vi "Wait for Control Panel Start.vi"(8 "error in (no error)":errorcluster, 10 "timeout in ms (-1)":i32=-1, 11 "Generic Controller in":refnum<class "Generic Plugin.lvclass">) -> (0 "error out":errorcluster, 2 "Timeout?":bool, 3 "Generic Controller out":refnum<class "Generic Plugin.lvclass">)   [LabVIEW 2020, in "Generic Plugin.lvclass"]
doc: "Wait for a message indicating that the control panel has started, or timeout if a value is given for the wait time."
uses:
  Generic Plugin.lvclass
  Generic Plugin.lvclass/Generic Plugin.ctl
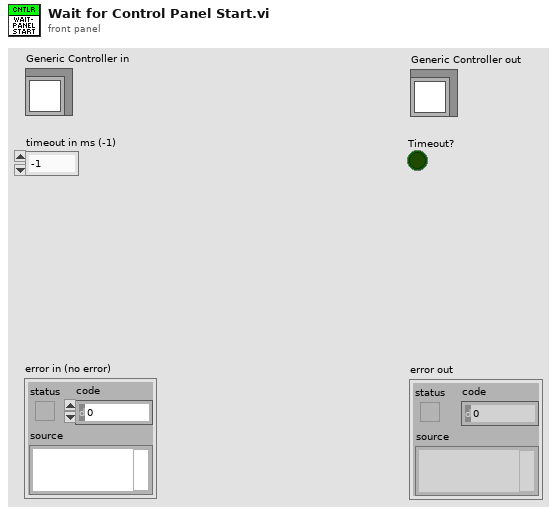
[diagram p1: front panel]
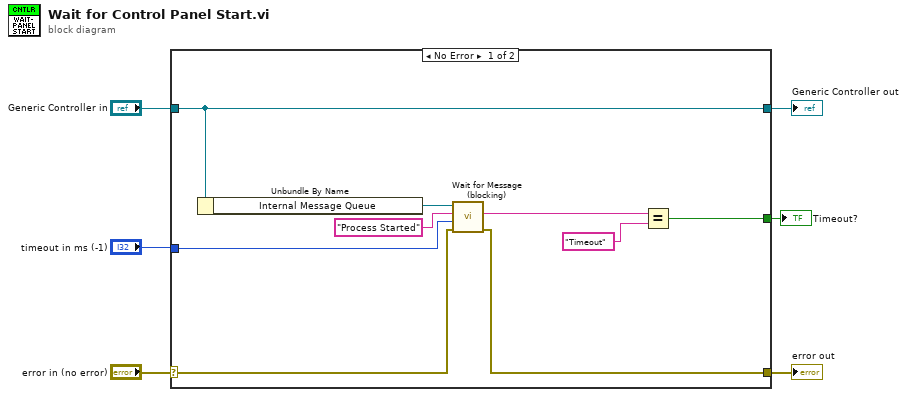
[diagram p0: block diagram]
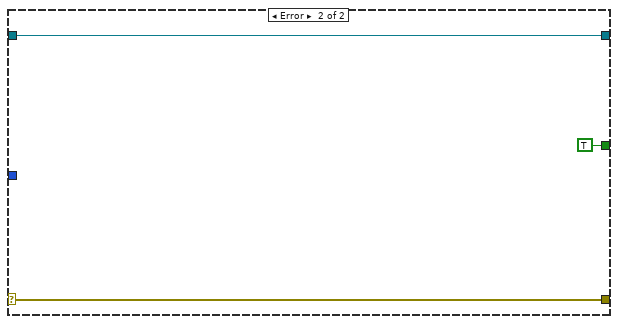
[diagram p2: hidden frame]
diagram:
  n1 = case shown="No Error" "error in (no error)" {
    selector: "error in (no error)" -> [w13 w18]
    tunnel: [w11 w18] -> w5
    tunnel: [w15 w17] -> w3
    tunnel: "Generic Controller in" -> [w15 w17]
    tunnel: "timeout in ms (-1)" -> [w10 _]
    tunnel: [w7 TRUE] -> w1
    frame No Error {
      n2 = Unbundle By Name(w15) -> ("Internal Message Queue"=w14:refnum<queue>)
      n3 = call "Wait for Message (blocking).vi"("error in (no error)"=w13, "timeout in ms (-1)"=w10, "Command"="Process Started", "Listening queue in"=w14) -> ("error out"=w11:errorcluster, "Message"=w9:string)  [unwired: 4 in, 2 out]
      n4 = Equal?(x=w9, y="Timeout") -> (x = y?=w7:bool)
    }
    frame Error {
    }
  }
  "error out" <- w5
  "Generic Controller out" <- w3
  "Timeout?" <- w1
